vi "Get Observables Values.vi"(8 "error in (no error)":errorcluster, 10 "Observables":string[](array[string]), 11 "Analysis Framework in":refnum<class "Analysis Framework.lvclass">) -> (0 "error out":errorcluster, 1 "Missing values":bool, 2 "Observables with values":T1[](array[typedef]), 3 "Analysis Framework out":refnum<class "Analysis Framework.lvclass">)   [LabVIEW 2020, in "TALOS.lvlib" / "Interfaces.lvlib" / "Analysis Framework.lvclass"]
uses:
  Analysis Framework.lvclass
  Run Utilities/Optimiser Cell/Name with value pair.ctl
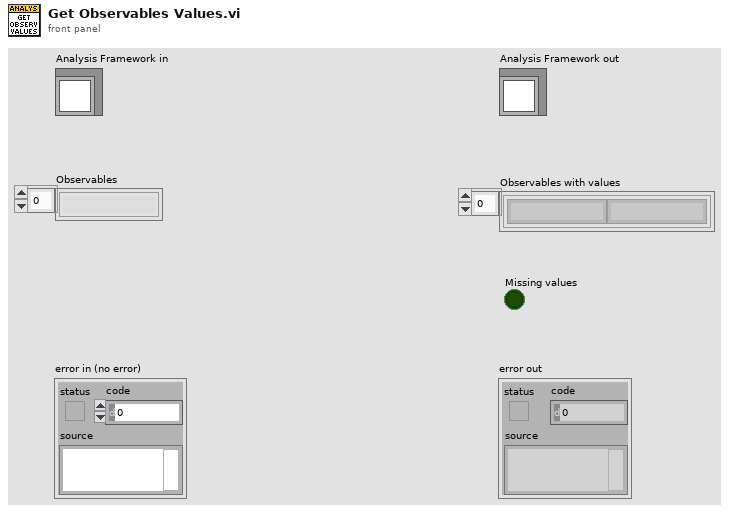
[diagram p1: front panel]
types:
  T1 = typedef "TALOS.lvlib/Interfaces.lvlib/Analysis Framework.lvclass/Name with value pair.ctl" = cluster{"Name":string, "Value":string}
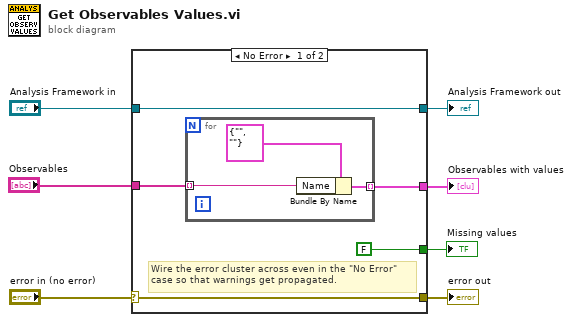
[diagram p0: block diagram]
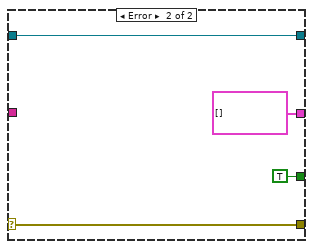
[diagram p2: hidden frame]
diagram:
  n1 = case shown="No Error" "error in (no error)" {
    selector: "error in (no error)" -> [w11 w19]
    tunnel: [w11 w19] -> w6
    tunnel: [w12 w18] -> w4
    tunnel: "Analysis Framework in" -> [w12 w18]
    tunnel: "Observables" -> [w10 _]
    tunnel: [w9 T1[] []] -> w2
    tunnel: [FALSE TRUE] -> w1
    frame No Error {
      # "Wire the error cluster across even in the \"No Error\"\ncase so that warnings get propagated."
      n2 = for {
        tunnel: w10 -> [w14] mode=indexing
        tunnel: [w13] -> w9 mode=indexing
        n3 = Bundle By Name(cluster=T1 {"Name"="", "Value"=""} ("Observable"), "Name"=w14) -> (w13:T1)
      }
    }
    frame Error {
    }
  }
  "error out" <- w6
  "Analysis Framework out" <- w4
  "Observables with values" <- w2
  "Missing values" <- w1
